vi "Register Subsystem.vi"(8 "error in (no error)":errorcluster, 9 "Subsystem Name (optional)":string, 10 "JKI SMO in":refnum<class "SMO.lvclass">) -> (0 "error out":errorcluster, 1 "Attribute.Identity":refnum<class "Attribute.Identity.lvclass">, 2 "JKI SMO out":refnum<class "SMO.lvclass">)   [LabVIEW 2013, in "Registry-SMO.lvclass"]
uses:
  Registry-SMO.lvclass
  SMO/SMO.lvclass
  Support/Attribute.Identity/Attribute.Identity.lvclass
  SMO_Info--Cluster.ctl
  Registry-SMO.lvclass/Registry-SMO.ctl
  Support/Attribute.Identity/Attribute.Identity.lvclass/Attribute.Identity.ctl
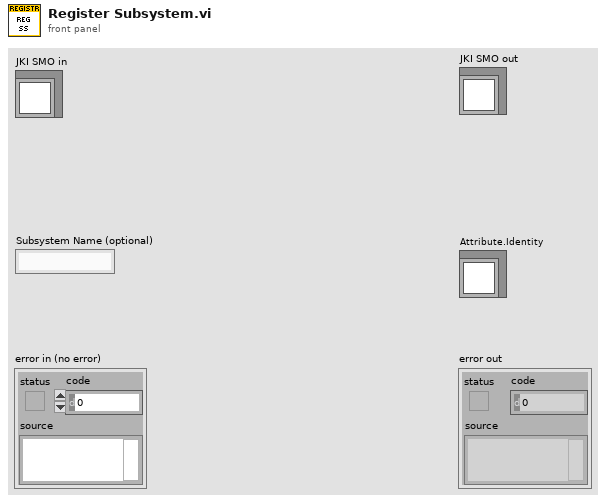
[diagram p1: front panel]
types:
  T1 = typedef "Registry-SMO.lvclass/SMO_Info--Cluster.ctl" = cluster{"Name":string, "Shared Resource":bool}
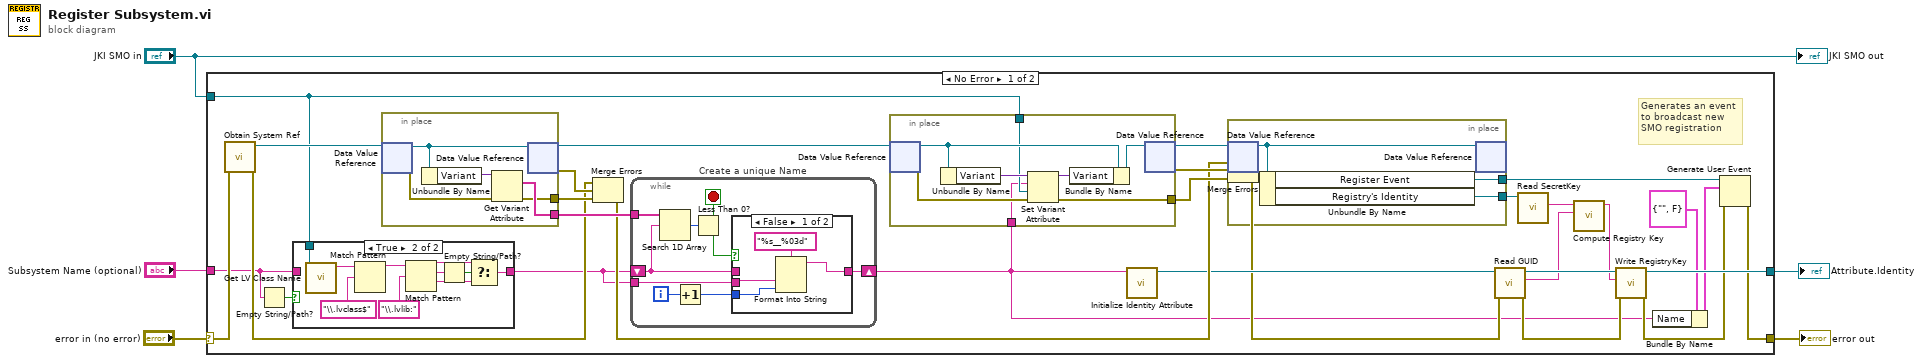
[diagram p0: block diagram]
diagram:
  n1 = case shown="No Error" "error in (no error)" {
    selector: "error in (no error)" -> [w33 w76]
    tunnel: [w9 w76] -> w4
    tunnel: "Subsystem Name (optional)" -> [w7 _]
    tunnel: "JKI SMO in" -> [w30 _]
    tunnel: [w22 _] -> w2
    frame No Error {
      # "Generates an event\nto broadcast new\nSMO registration"
      n2 = call "Obtain System Ref.vi"("error in (no error)"=w33) -> ("error out"=w25:errorcluster, "JKI SMO System"=w32:refnum<data-value>)  [unwired: 9 in]
      n3 = Empty String/Path?(string/path=w7) -> (empty?=w31:bool)
      n4 = case shown="True" w31 {
        tunnel: w7 -> [w52 _]
        tunnel: [w52 w53] -> w6
        tunnel: w30 -> [_ w62]
        frame False {
        }
        frame True {
          n5 = call <vilib>:"Get LV Class Name.vi"("object"=w62) -> ("class name"=w54:string)  [unwired: 9 in, 1 out]
          n6 = Match Pattern(string=w54, regular expression="\\.lvclass$") -> (before substring=w60:string)  [unwired: 1 in, 3 out]
          n7 = Match Pattern(string=w60, regular expression="\\.lvlib:") -> (before substring=w56:string, match substring=w58:string, after substring=w55:string)  [unwired: 1 in, 1 out]
          n8 = Empty String/Path?(string/path=w58) -> (empty?=w57:bool)
          n9 = Select(t=w56, s=w57, f=w55) -> (s? t:f=w53:string)
        }
      }
      n10 = in-place {
        in-place-border: [w64] -> w29
        in-place-border: [w63] -> w26
        n11 = in-place-dvr #1(w32) -> (w67:refnum<class "Registry-SMO.lvclass">, w65:errorcluster)
        n12 = Unbundle By Name(w67) -> ("Variant"=w66:variant)
        n13 = Get Variant Attribute(Variant=w66, error in=w65) -> (names=w64:string[], error out=w63:errorcluster)  [unwired: 2 in, 2 out]
        n14 = in-place-dvr #1(w67) -> (w28:refnum<data-value>, w27:errorcluster)
      }
      n15 = Merge Errors(w25, w27, w26) -> (w24:errorcluster)
      n16 = while "Create a unique Name" {
        tunnel: w29 -> [w46]
        shift-right: [w42] -> w8
        shift-left: w6 -> [w43]
        tunnel: w6 -> [w41]
        i -> [w40]
        stop <- w44 stop-if-true
        n17 = Search 1D Array(1D array=w46, element=w43) -> (index of element=w45:i32)  [unwired: 1 in]
        n18 = Increment(x=w40) -> (x+1=w39:i32)
        n19 = Less Than 0?(x=w45) -> (x < 0?=w44:bool)
        n20 = case shown="False" w44 {
          tunnel: w43 -> [_ w51]
          tunnel: [w49 w51] -> w42
          tunnel: w41 -> [w50 _]
          tunnel: w39 -> [w48 _]
          frame False {
            n21 = Format Into String(format string="%s__%03d", w50, w48) -> (resulting string=w49:string)  [unwired: 2 in, 1 out]
          }
          frame True {
            # "Name is unique"
          }
        }
      }
      n22 = in-place {
        in-place-border: w30 -> [w72]
        in-place-border: [w70] -> w34
        in-place-border: w8 -> [w68]
        n23 = in-place-dvr #2(w28) -> (w75:refnum<class "Registry-SMO.lvclass">, w69:errorcluster)
        n24 = Unbundle By Name(w75) -> ("Variant"=w73:variant)
        n25 = Set Variant Attribute(Variant=w73, name=w68, value=w72, error in=w69) -> (Variant out=w71:variant, error out=w70:errorcluster)  [unwired: 1 out]
        n26 = Bundle By Name(cluster=w75, "Variant"=w71) -> (w74:refnum<class "Registry-SMO.lvclass">)
        n27 = in-place-dvr #2(w74) -> (w23:refnum<data-value>, w35:errorcluster)
      }
      n28 = call "Initialize Identity Attribute.vi"("Name"=w8) -> ("Attribute.Identity"=w21:refnum<class "Attribute.Identity.lvclass">)  [unwired: 10 in]
      n29 = in-place {
        in-place-border: [w37] -> w19
        in-place-border: [w36] -> w13
        n30 = in-place-dvr #3(w23) -> (w38:refnum<class "Registry-SMO.lvclass">)  [unwired: 1 out]
        n31 = Unbundle By Name(w38) -> ("Register Event"=w36:refnum<user-event>, "Registry's Identity"=w37:refnum<class "Attribute.Identity.lvclass">)
        n32 = in-place-dvr #3(w38) -> ()  [unwired: 2 out]
      }
      n33 = Merge Errors(w24, w35, w34) -> (w15:errorcluster)
      n34 = call "Read GUID.vi"("error in (no error)"=w15, "Attribute.Identity in"=w21) -> ("error out"=w14:errorcluster, "GUID"=w17:string, "Attribute.Identity out"=w20:refnum<class "Attribute.Identity.lvclass">)  [unwired: 7 in]
      n35 = call "Read SecretKey.vi"("Attribute.Identity in"=w19) -> ("SecretKey"=w18:string)  [unwired: 8 in, 2 out]
      n36 = call "Compute Registry Key.vi"("SMO GUID"=w17, "Registry's SecretKey"=w18) -> ("Registry Key"=w16:string)  [unwired: 9 in]
      n37 = call "Write RegistryKey.vi"("error in (no error)"=w14, "RegistryKey"=w16, "Attribute.Identity in"=w20) -> ("error out"=w10:errorcluster, "Attribute.Identity out"=w22:refnum<class "Attribute.Identity.lvclass">)  [unwired: 7 in]
      n38 = Bundle By Name(cluster=T1 {"Name"="", "Shared Resource"=FALSE} ("Cluster"), "Name"=w8) -> (w11:T1)
      n39 = Generate User Event(user event=w13, event data cluster=w11, error in=w10) -> (error out=w9:errorcluster)  [unwired: 1 in, 1 out]
    }
    frame Error {
    }
  }
  "error out" <- w4
  "Attribute.Identity" <- w2
  "JKI SMO out" <- "JKI SMO in"
